vi "test Getting Owned String Handle.vi"(8 "error in (no error)":errorcluster, 11 "TestCase in":refnum<class "String Tests.lvclass">=refnum) -> (0 "error out":errorcluster, 3 "TestCase out":refnum<class "String Tests.lvclass">)   [LabVIEW 2023, in "String Tests.lvclass"]
uses:
  String Tests.lvclass
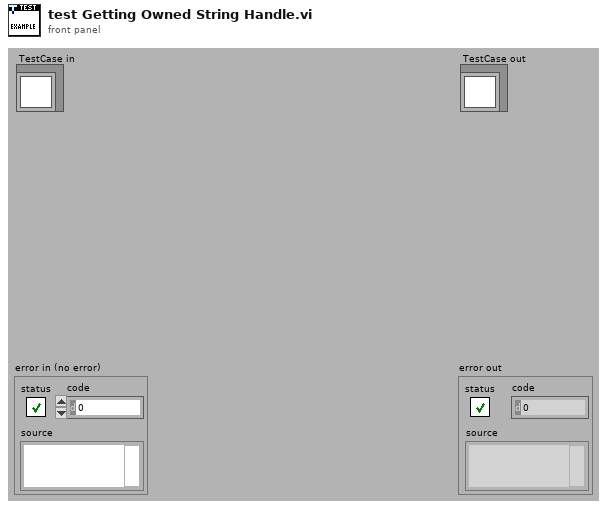
[diagram p1: front panel]
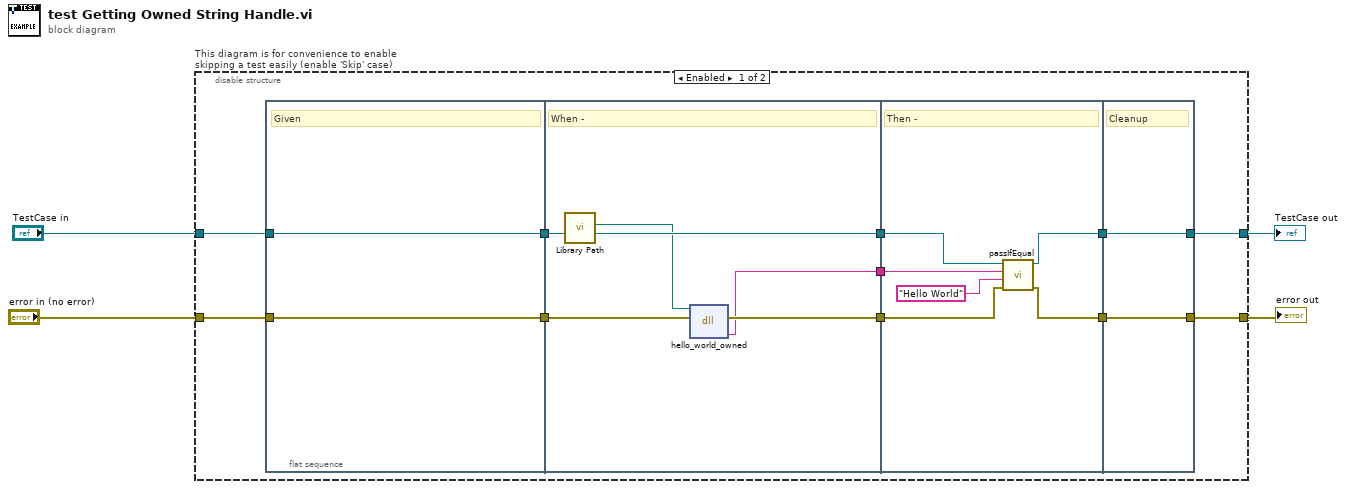
[diagram p0: block diagram]
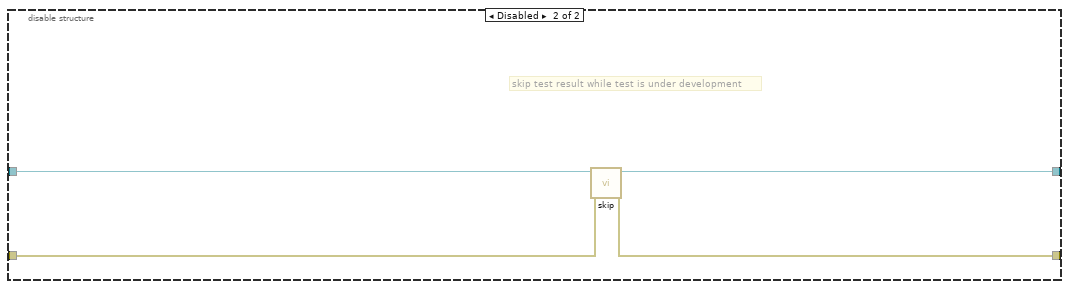
[diagram p2: hidden frame]
diagram:
  n1 = disable-structure "This diagram is for convenience to enable skipping a test easily (enable 'Skip' case)" shown="Enabled" {
    disable-tunnel: "TestCase in" -> [w9 w34]
    disable-tunnel: [w7 w32] -> w1
    disable-tunnel: [w6 w33] -> w3
    disable-tunnel: "error in (no error)" -> [w8 w31]
    frame Enabled {
      n2 = flat-sequence {
        tunnel: w8 -> [w16]
        tunnel: w9 -> [w17]
        tunnel: [w17] -> w15
        tunnel: [w16] -> w14
        tunnel: [w22] -> w13
        tunnel: [w20] -> w12
        tunnel: w15 -> [w22]
        tunnel: w14 -> [w19]
        tunnel: [w18] -> w5
        tunnel: [w27] -> w11
        tunnel: [w25] -> w10
        tunnel: w13 -> [w28]
        tunnel: w12 -> [w26]
        tunnel: w5 -> [w24]
        tunnel: [w29] -> w6
        tunnel: [w30] -> w7
        tunnel: w11 -> [w30]
        tunnel: w10 -> [w29]
        frame #0 {
          # "Given"
        }
        frame #1 {
          # "When -"
          n3 = call "Library Path.vi"() -> ("Library Path"=w21:path)  [unwired: 11 in]
          n4 = dll-call lib="C:/Users/JamesMcNally/Documents/RustInterop/Rust-LabVIEW-Interop/target/debug/labview_test_library.dll" fn="hello_world_owned"(path in=w21, error in=w19) -> (error out=w20:errorcluster, "string"=w18:string)  [unwired: 3 in, 1 out]
        }
        frame #2 {
          # "Then -"
          n5 = call-dynamic "passIfEqual.vi"("error in (no error)"=w26, "y"="Hello World" ("string"), "x"=w24, "TestCase in"=w28) -> ("error out"=w25:errorcluster, "TestCase out"=w27:refnum<class "String Tests.lvclass">)  [unwired: 6 in]
        }
        frame #3 {
          # "Cleanup"
        }
      }
    }
    frame Disabled {
      # "skip test result while test is under development"
      n6 = call <vilib>:"skip.vi"("error in (no error)"=w31, "TestCase in"=w34) -> ("error out"=w33:errorcluster, "TestCase out"=w32:refnum<class "String Tests.lvclass">)  [unwired: 8 in]
    }
  }
  "error out" <- w3
  "TestCase out" <- w1
